vi "GL_TempDspl.vi"() -> ()   [LabVIEW 2024]
panel:
  out "TEMPERATURE\nDisplay":dbl min=0.0 max=5000.0 format="%.4f"
  out "unit":enum16{"K", "Ohms", "C", "F"}(ring)
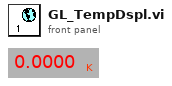
[diagram p1: front panel]
diagram:
